vi "Write Curves.vi"(8 "error in (no error)":errorcluster, 10 "Curves":T1[](array[typedef]) {"Points"."Y" format="%.2f"; "Points"."X" format="%.2f"}, 11 "EdgeDetectionProcessor in":refnum<class "EdgeDetectionProcessor.lvclass">) -> (0 "error out":errorcluster, 3 "EdgeDetectionProcessor out":refnum<class "EdgeDetectionProcessor.lvclass">)   [LabVIEW 2018, in "EdgeDetectionProcessor.lvclass"]
uses:
  EdgeDetectionProcessor.lvclass
  <vilib>/vision/Analysis.llb/IMAQ ExtractCurvesCurve.ctl
  EdgeDetectionProcessor.lvclass/EdgeDetectionProcessor.ctl
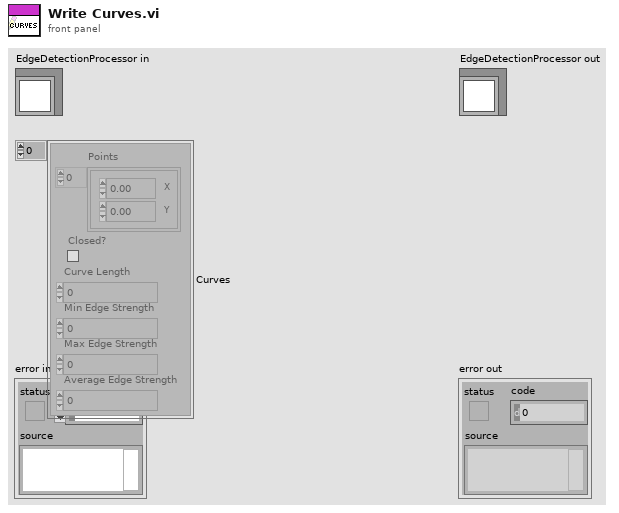
[diagram p1: front panel]
types:
  T1 = typedef "IMAQ ExtractCurvesCurve.ctl" = cluster{"Points":cluster{"X":dbl, "Y":dbl}[], "Closed?":bool, "Curve Length":dbl, "Min Edge Strength":dbl, "Max Edge Strength":dbl, "Average Edge Strength":dbl}
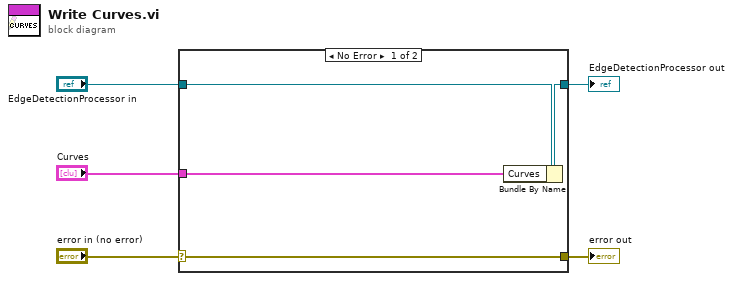
[diagram p0: block diagram]
diagram:
  n1 = case shown="No Error" "error in (no error)" {
    selector: "error in (no error)" -> [w9 w10]
    tunnel: [w9 w10] -> w4
    tunnel: [w7 w11] -> w2
    tunnel: "EdgeDetectionProcessor in" -> [w8 w11]
    tunnel: "Curves" -> [w6 _]
    frame No Error {
      n2 = Bundle By Name(cluster=w8, "Curves"=w6) -> (w7:refnum<class "EdgeDetectionProcessor.lvclass">)
    }
    frame Error {
    }
  }
  "error out" <- w4
  "EdgeDetectionProcessor out" <- w2
